vi "Do[Core].vi"(0 "ControlAction in":refnum<class "GetSubPanelVI.lvclass">, 5 "Ctl Refnum in":refnum<vi>, 11 "error in (no error)":errorcluster) -> (4 "ControlAction out":refnum<class "GetSubPanelVI.lvclass">, 6 "Ctl Refnum out":refnum<vi>, 15 "error out":errorcluster)   [LabVIEW 2016, in "GetSubPanelVI.lvclass"]
uses:
  GetSubPanelVI.lvclass
  GetSubPanelVI.lvclass/GetSubPanelVI.ctl
  VIActionBase/ControlActionBase.lvclass
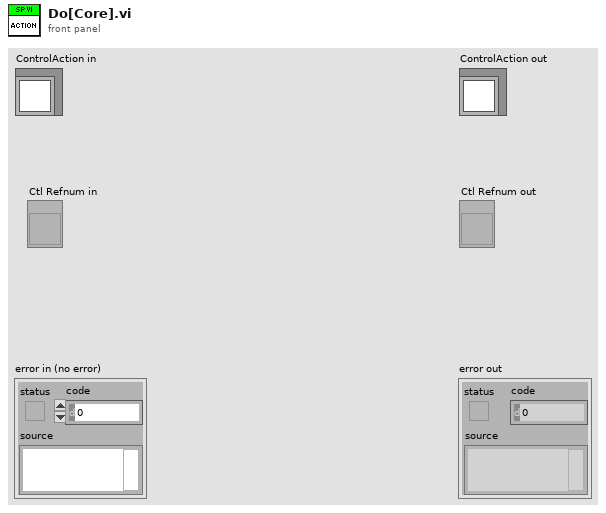
[diagram p1: front panel]
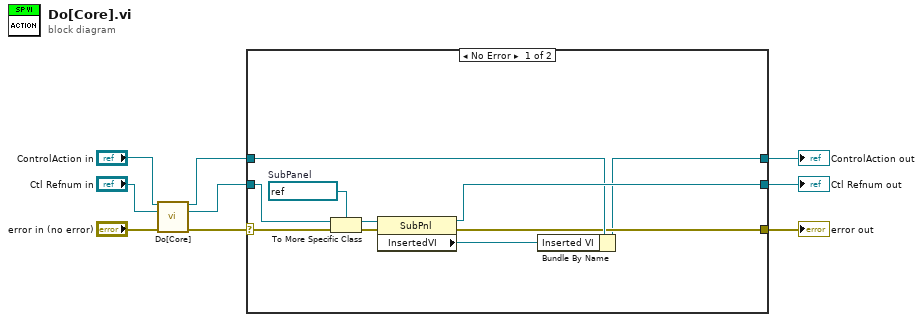
[diagram p0: block diagram]
diagram:
  n1 = call-parent "Do[Core].vi"("ControlAction in"="ControlAction in", "Ctl Refnum in"="Ctl Refnum in", "error in (no error)"="error in (no error)") -> ("ControlAction out"=w1:refnum<class "GetSubPanelVI.lvclass">, "Ctl Refnum out"=w5:refnum<vi>, "error out"=w4:errorcluster)  [unwired: 10 in]
  n2 = case shown="No Error" w4 {
    selector: w4 -> [w17 w22]
    tunnel: [w16 w22] -> w8
    tunnel: [w19 w21] -> w9
    tunnel: [w11 w20] -> w7
    tunnel: w5 -> [w14 w21]
    tunnel: w1 -> [w18 w20]
    frame No Error {
      w12 = refnum<vi> refnum  # SubPanel
      n3 = To More Specific Class(target class=w12, reference=w14, error in=w17) -> (specific class reference=w13:refnum<vi>, error out=w15:errorcluster)
      n4 = property class="SubPnl"(reference=w13, error in=w15) -> (reference out=w19:refnum<vi>, error out=w16:errorcluster, "InsertedVI"=w10:refnum<vi>)
      n5 = Bundle By Name(cluster=w18, "Inserted VI"=w10) -> (w11:refnum<class "GetSubPanelVI.lvclass">)
    }
    frame Error {
    }
  }
  "error out" <- w8
  "ControlAction out" <- w7
  "Ctl Refnum out" <- w9
